vi "CFTS-Manual Path.vi"() -> (0 "Path":path)   [LabVIEW 2020]
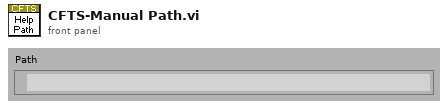
[diagram p1: front panel]
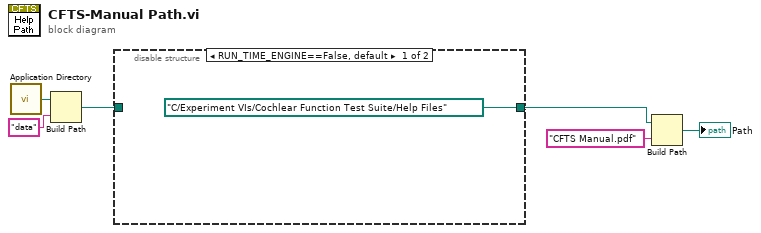
[diagram p0: block diagram]
diagram:
  n1 = call <vilib>:"Application Directory.vi"() -> ("Application Directory"=w3:path)
  n2 = Build Path(base path=w3, name or relative path="data") -> (appended path=w1:path)
  n3 = disable-structure shown="RUN_TIME_ENGINE==False, default" {
    disable-tunnel: [path "C:/Experiment VIs/Cochlear Function Test Suite/Help Files" ("acrobat document") w8] -> w4
    disable-tunnel: w1 -> [_ w8]
    frame condition #0 (active) {
    }
    frame condition #1 {
    }
  }
  n4 = Build Path(base path=w4, name or relative path="CFTS Manual.pdf") -> (appended path=→"Path":path)
